vi "Conditionning - Auto Truncate wForms.vi"(0 "reference in":refnum<class "GSwFormDSP.lvclass">, 5 "error in (no error)":errorcluster, 7 "Auto Cut Signals":T1={"Ref Channel"=-1, "Trigger Amplitude"=0.0, "Pre Trigger Length (sec)"=0.0, "Duration (sec)"=0.0}) -> (11 "actual start samples/time":dbl format="%_8f", 13 "actual duration":dbl format="%0.2f", 14 "reference in":refnum<class "GSwFormDSP.lvclass">, 19 "error out":errorcluster)   [LabVIEW 2020, in "GSwFormDSP.lvclass"]
uses:
  GSwFormDSP.lvclass
  <vilib>/measure/mamon.llb/Trigger Detection for 1 Channel.vi
  <vilib>/measure/NI_MAPro.lvlib
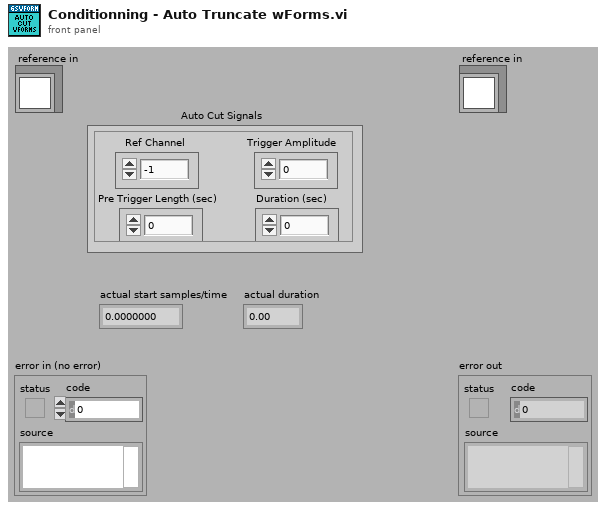
[diagram p1: front panel]
types:
  T1 = cluster{"Ref Channel":i32, "Trigger Amplitude":dbl, "Pre Trigger Length (sec)":dbl, "Duration (sec)":dbl}
  T2 = enum16{"KEEP the specified Segment", "DELETE the specified Segment"}
  T3 = typedef "GSwFormDSP.lvclass/ObjectAttributesRef.ctl" = refnum<data-value>
  T4 = typedef "GSwFormDSP.lvclass/ObjectAttributes.ctl" = cluster{"Wform Ref":refnum<data-value>, "Nb Signals":i32, "Spectral Function Parameters":T5, "FFT":waveform(cdb)[], "Nb FFT":i32, "Nb Averages":i32[], "Reference Indexes":i32[], "Response Indexes":i32[], "Coherence":waveform(dbl)[], "TDF Parameters":T7, "DAQ":cluster{"Duration (sec)":dbl, "Buffer Size (Samples)":i32, "Offset (Samples)":i32}, "Filter Impulse Response (TDF)":waveform(dbl), "Sound Playback":T8}
  T5 = typedef "GSwFormDSP.lvclass/Spectral Parameters.ctl" = cluster{"Frequency resolution (Hz)":dbl, "Overlap":dbl, "Window":T6}
  T6 = typedef "NI_AALPro.lvlib/windowTd.ctl" = u32
  T7 = typedef "GSwFormDSP.lvclass/TDF Parameters.ctl" = cluster{"Filter":enum32{"Lowpass", "Highpass", "Bandpass", "Bandstop"}, "Type:":enum16{"Butterworth", "Chebyshev", "Inv Chebyshev", "Elliptic", "Bessel"}, "LP cutoff freq":dbl, "HP cutoff freq":dbl, "Order":i32, "passband ripple (dB)":dbl, "stopband attenuation (dB)":dbl, "Phaseless Filter":bool, "Include Fade IN and OUT":bool}
  T8 = typedef "GSwFormDSP.lvclass/Sound Playback.ctl" = cluster{"Timer start (ms)":u32, "task ID":T9, "Cursor Init Location (s)":dbl, "SC Volume":dbl}
  T9 = typedef "Sound Output Task ID.ctl" = u32
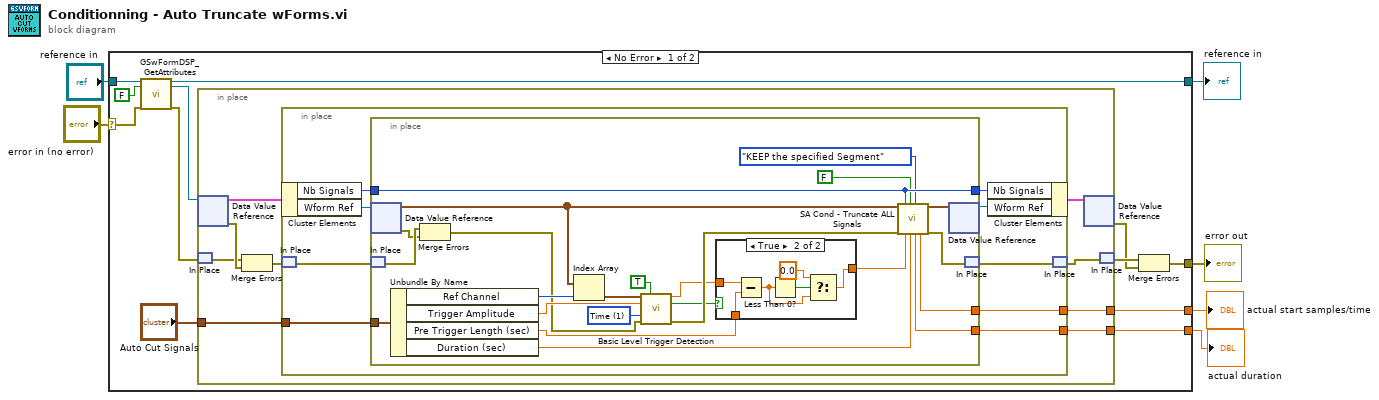
[diagram p0: block diagram]
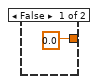
[diagram p2: hidden frame]
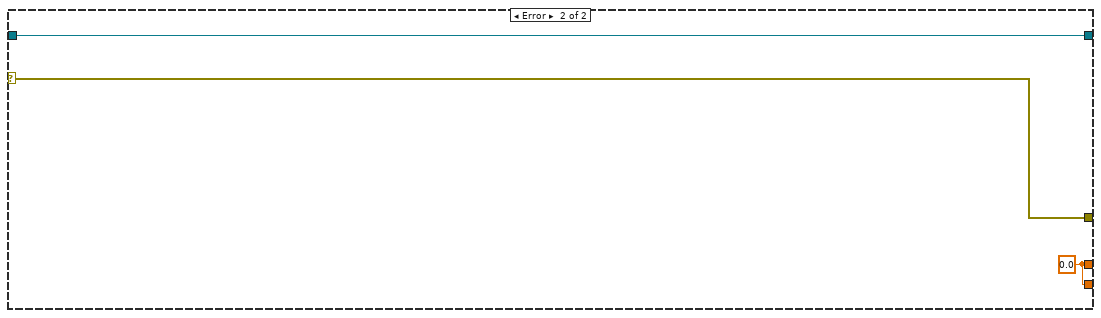
[diagram p3: hidden frame]
diagram:
  n1 = case shown="No Error" "error in (no error)" {
    selector: "error in (no error)" -> [w15 w69]
    tunnel: [w18 w69] -> w5
    tunnel: [w13 w68] -> w3
    tunnel: "reference in" -> [w16 w68]
    tunnel: [w9 w67] -> w2
    tunnel: [w8 w67] -> w1
    frame No Error {
      n2 = call "GSwFormDSP_GetAttributes.vi"("reference in"=w16, "return data? (T)"=FALSE, "error in (no error)"=w15) -> ("reference out"=w13:refnum<class "GSwFormDSP.lvclass">, "attributes ref"=w14:T3, "error out"=w12:errorcluster)  [unwired: 13 in, 1 out]
      n3 = in-place {
        in-place-border: [w21] -> w9
        in-place-border: [w20] -> w8
        in-place-border: "Auto Cut Signals" -> [w19]
        n4 = in-place-dvr #1(w14) -> (w25:T4, w27:errorcluster)
        n5 = in-place-match #2(w12) -> (w26:errorcluster)
        n6 = Merge Errors(w26, w27) -> (w24:errorcluster)
        n7 = in-place {
          in-place-border: [w31] -> w21
          in-place-border: [w30] -> w20
          in-place-border: w19 -> [w28]
          n8 = in-place-cluster #3(w25) -> ("Nb Signals"=w32:i32, "Wform Ref"=w36:refnum<data-value>)
          n9 = in-place-match #4(w24) -> (w34:errorcluster)
          n10 = in-place {
            in-place-border: w32 -> [w53]
            in-place-border: [w55] -> w31
            in-place-border: [w54] -> w30
            in-place-border: [w53] -> w29
            in-place-border: w28 -> [w48]
            w43 = u16 1 items=["Index", "Time"] ("location mode")
            n11 = in-place-dvr #5(w36) -> (w50:waveform(dbl)[], w57:errorcluster)
            n12 = in-place-match #6(w34) -> (w58:errorcluster)
            n13 = Unbundle By Name(w48) -> ("Ref Channel"=w49:i32, "Trigger Amplitude"=w44:dbl, "Pre Trigger Length (sec)"=w38:dbl, "Duration (sec)"=w47:dbl)
            n14 = Merge Errors(w58, w57) -> (w42:errorcluster)
            n15 = Index Array(array=w50, index=w49) -> (element=w46:waveform(dbl))
            n16 = call-poly <vilib>:"Basic Level Trigger Detection.vi"("signal in"=w46, "reset"=TRUE, "level"=w44, "location mode"=w43, "error in (no error)"=w42) -> ("trigger location"=w39:dbl, "trigger detected?"=w40:bool, "error out"=w41:errorcluster)  [unwired: 8 in]
            n17 = case shown="True" w40 {
              tunnel: w39 -> [_ w66]
              tunnel: w38 -> [_ w65]
              tunnel: [0.0 w63] -> w37
              frame False {
              }
              frame True {
                n18 = Subtract(x=w66, y=w65) -> (x-y=w62:dbl)
                n19 = Less Than 0?(x=w62) -> (x < 0?=w64:bool)
                n20 = Select(t=0.0, s=w64, f=w62) -> (s? t:f=w63:dbl)
              }
            }
            n21 = call "SA Cond - Truncate ALL Signals.vi"("wForm IN"=w50, "error in (no error)"=w41, "Nb Signals"=w53, "Start (sec)"=w37, "Anotate Signal Name"=FALSE, "Duration (sec)"=w47, "Cut Option"=T2."KEEP the specified Segment") -> ("actual duration"=w54:dbl, "actual start samples/time"=w55:dbl, "wForm OUT"=w59:waveform(dbl)[], "error out"=w56:errorcluster)  [unwired: 9 in]
            n22 = in-place-dvr #5(w59) -> (w35:refnum<data-value>)  [unwired: 1 out]
            n23 = in-place-match #6(w56) -> (w33:errorcluster)
          }
          n24 = in-place-cluster #3("Nb Signals"=w29, "Wform Ref"=w35) -> (w23:T4)
          n25 = in-place-match #4(w33) -> (w22:errorcluster)
        }
        n26 = in-place-dvr #1(w23) -> (w10:errorcluster)  [unwired: 1 out]
        n27 = in-place-match #2(w22) -> (w11:errorcluster)
      }
      n28 = Merge Errors(w11, w10) -> (w18:errorcluster)
    }
    frame Error {
      w67 = 0.0 ("actual start samples/time")
    }
  }
  "error out" <- w5
  "reference in" <- w3
  "actual start samples/time" <- w2
  "actual duration" <- w1
